vi "ReadPointDataFromNewString.vi"(8 "error in (no error)":errorcluster, 9 "New String":string) -> (0 "error out":errorcluster, 1 "X index":dbl, 2 "Y val":dbl, 3 "X val":dbl, 4 "Z/F(x)":dbl, 5 "Y Index":dbl)   [LabVIEW 2023]
uses:
  StringFormatGlobals.vi
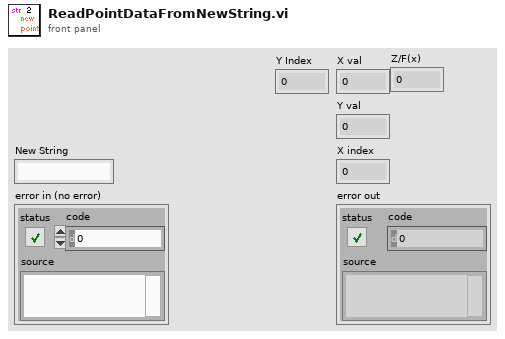
[diagram p1: front panel]
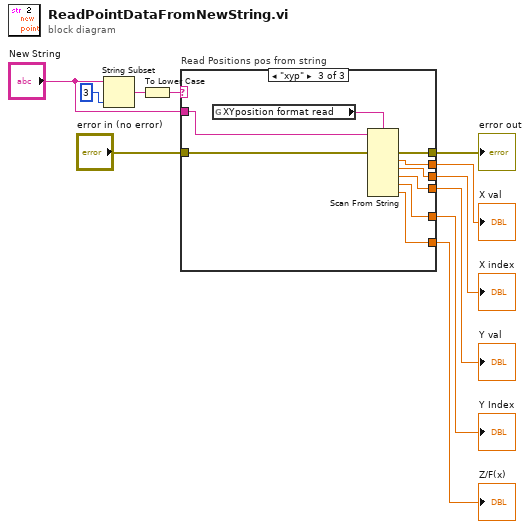
[diagram p0: block diagram]
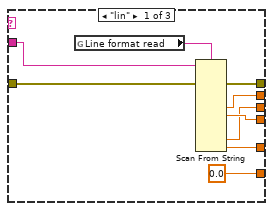
[diagram p2: hidden frame]
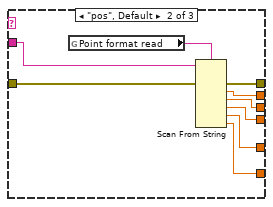
[diagram p3: hidden frame]
diagram:
  n1 = String Subset(string="New String", length (rest)=3 ("length (rest)")) -> (substring=w5:string)  [unwired: 1 in]
  n2 = To Lower Case(string=w5) -> (all lower case string=w2:string)
  n3 = case "Read Positions pos from string" shown="\"xyp\"" w2 {
    tunnel: "New String" -> [w20 w29 w38]
    tunnel: [w17 w28 w37] -> w10
    tunnel: [w16 w27 w36] -> w11
    tunnel: [w15 w26 w35] -> w6
    tunnel: [w14 w25 w34] -> w9
    tunnel: "error in (no error)" -> [w19 w24 w33]
    tunnel: [w18 w23 w32] -> w8
    tunnel: [0.0 w21 w30] -> w1
    frame "lin" {
      n4 = global read "StringFormatGlobals.vi" "Line format read"() -> (w13:string)
      n5 = Scan From String(format string=w13, input string=w20, error in=w19) -> (error out=w18:errorcluster, output 3=w17:dbl, output 4=w16:dbl, output 7=w15:dbl, output 8=w14:dbl)  [unwired: 13 in, 2 out]
    }
    frame "pos", Default {
      n6 = global read "StringFormatGlobals.vi" "Point format read"() -> (w22:string)
      n7 = Scan From String(format string=w22, input string=w29, error in=w24) -> (error out=w23:errorcluster, output 1=w28:dbl, output 2=w26:dbl, output 3=w27:dbl, output 4=w25:dbl, output 5=w21:dbl)  [unwired: 6 in, 2 out]
    }
    frame "xyp" {
      n8 = global read "StringFormatGlobals.vi" "XYposition format read"() -> (w31:string)
      n9 = Scan From String(format string=w31, input string=w38, error in=w33) -> (error out=w32:errorcluster, output 1=w37:dbl, output 2=w35:dbl, output 3=w36:dbl, output 4=w34:dbl, output 5=w30:dbl)  [unwired: 6 in, 2 out]
    }
  }
  "Y val" <- w11
  "X val" <- w10
  "Y Index" <- w9
  "X index" <- w6
  "error out" <- w8
  "Z/F(x)" <- w1
